vi "GetAllNames.vi"(8 "error in (no error)":errorcluster) -> (0 "error out":errorcluster, 2 "Keys":string[](array[string]))   [LabVIEW 2024, in "LogSingleton.lvlib"]
uses:
  LogSingleton.lvlib
  fgvCommands.ctl
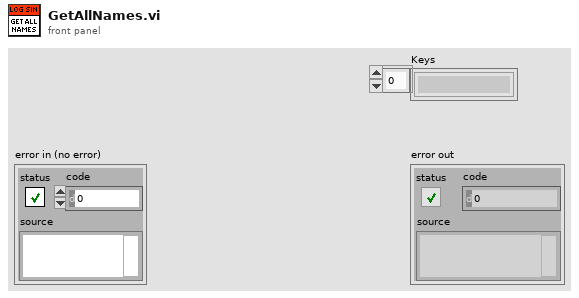
[diagram p1: front panel]
types:
  T1 = typedef "LogSingleton.lvlib/fgvCommands.ctl" = enum16{"Add", "Get", "GetAllKeys", "Remove"}
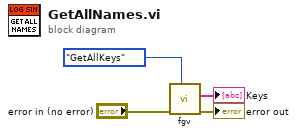
[diagram p0: block diagram]
diagram:
  n1 = call "fgv.vi"("fgv command"=fgvCommands."GetAllKeys", "error in (no error)"="error in (no error)") -> ("error out"=→"error out":errorcluster, "Keys"=→"Keys":string[])  [unwired: 7 in, 1 out]
